vi "base64_decode.vi"(11 "base64":string) -> (3 "string":string)   [LabVIEW 2018, in "hashlib.lvlib"]
doc: "Decodes the <b>Base64</b> data from the <b>base64</b> string input.\n\nRFC 4648\n\nCreated by: Ryan Pacini"
uses:
  hashlib.lvlib
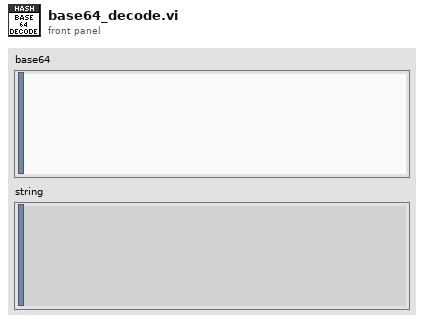
[diagram p1: front panel]
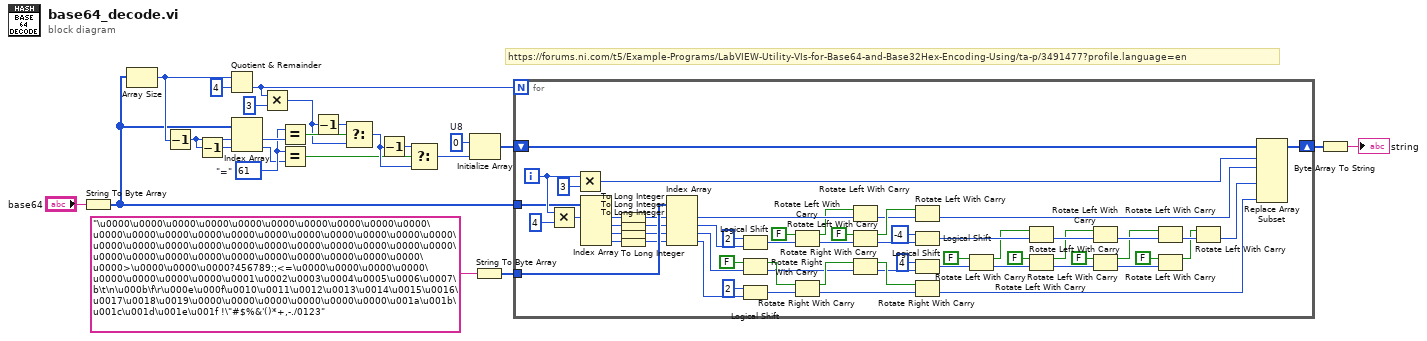
[diagram p0: block diagram]
diagram:
  w11 = u8 61  # "="
  w21 = u8 0  # U8
  # "https://forums.ni.com/t5/Example-Programs/LabVIEW-Utility-VIs-for-Base64-and-Base32Hex-Encoding-Using/ta-p/3491477?profile.language=en"
  n1 = String To Byte Array(string="base64") -> (unsigned byte array=w1:u8[])
  n2 = Array Size(array=w1) -> (size(s)=w18:i32)
  n3 = Decrement(x=w18) -> (x-1=w14:i32)
  n4 = Decrement(x=w14) -> (x-1=w13:i32)
  n5 = Quotient & Remainder(x=w18, y=4) -> (floor(x/y)=w2:i32)  [unwired: 1 out]
  n6 = Index Array(array=w1, index #1=w14, index #2=w13) -> (element #1=w12:u8, element #2=w10:u8)
  n7 = Multiply(x=w2, y=3) -> (x*y=w8:i32)
  n8 = Equal?(x=w11, y=w12) -> (x = y?=w9:bool)
  n9 = Equal?(x=w11, y=w10) -> (x = y?=w4:bool)
  n10 = Decrement(x=w8) -> (x-1=w7:i32)
  n11 = Select(t=w7, s=w9, f=w8) -> (s? t:f=w5:i32)
  n12 = Decrement(x=w5) -> (x-1=w6:i32)
  n13 = Select(t=w6, s=w4, f=w5) -> (s? t:f=w3:i32)
  n14 = Initialize Array(w21, w3) -> (w20:u8[])
  n15 = String To Byte Array(string="\u0000\u0000\u0000\u0000\u0000\u0000\u0000\u0000\u0000\u0000\u0000\u0000\u0000\u0000\u0000\u0000\u0000\u0000\u0000\u0000\u0000\u0000\u0000\u0000\u0000\u0000\u0000\u0000\u0000\u0000\u0000\u0000\u0000\u0000\u0000\u0000\u0000\u0000\u0000\u0000\u0000\u0000\u0000>\u0000\u0000\u0000?456789:;<=\u0000\u0000\u0000\u0000\u0000\u0000\u0000\u0000\u0001\u0002\u0003\u0004\u0005\u0006\u0007\b\t\n\u000b\f\r\u000e\u000f\u0010\u0011\u0012\u0013\u0014\u0015\u0016\u0017\u0018\u0019\u0000\u0000\u0000\u0000\u0000\u0000\u001a\u001b\u001c\u001d\u001e\u001f !\"#$%&'()*+,-./0123") -> (unsigned byte array=w15:u8[])
  n16 = for {
    N: w2 -> [_]
    shift-right: [w37] -> w17
    shift-left: w20 -> [w36]
    tunnel: w1 -> [w79]
    tunnel: w15 -> [w29]
    i -> [w82]
    n17 = Multiply(x=w82, y=4) -> (x*y=w80:i32)
    n18 = Multiply(x=w82, y=3) -> (x*y=w83:i32)
    n19 = Index Array(array=w79, index #1=w80) -> (element #1=w78:u8, element #2=w77:u8, element #3=w76:u8, element #4=w75:u8)  [unwired: 3 in]
    n20 = To Long Integer(number=w78) -> (32bit integer=w28:i32)
    n21 = To Long Integer(number=w77) -> (32bit integer=w27:i32)
    n22 = To Long Integer(number=w76) -> (32bit integer=w26:i32)
    n23 = To Long Integer(number=w75) -> (32bit integer=w25:i32)
    n24 = Index Array(array=w29, index #1=w28, index #2=w27, index #3=w26, index #4=w25) -> (element #1=w74:u8, element #2=w72:u8, element #3=w58:u8, element #4=w59:u8)
    n25 = Logical Shift(y=i16 2, x=w72) -> (x << y=w71:u8)
    n26 = Rotate Right With Carry(2:w58, 3:FALSE ("carry")) -> (0:w55:u8, 1:w57:bool)
    n27 = Logical Shift(y=i16 2, x=w59) -> (x << y=w60:u8)
    n28 = Rotate Left With Carry(2:w71, 3:FALSE ("carry")) -> (0:w68:u8, 1:w67:bool)
    n29 = Rotate Right With Carry(2:w60, 3:w57) -> (0:w53:u8, 1:w56:bool)
    n30 = Rotate Left With Carry(2:w74, 3:w67) -> (0:w65:u8)  [unwired: 1 out]
    n31 = Rotate Left With Carry(2:w68, 3:FALSE ("carry")) -> (0:w62:u8, 1:w66:bool)
    n32 = Rotate Right With Carry(2:w55, 3:w56) -> (0:w46:u8, 1:w54:bool)
    n33 = Rotate Left With Carry(2:w65, 3:w66) -> (0:w64:u8)  [unwired: 1 out]
    n34 = Logical Shift(y=i16 -4, x=w62) -> (x << y=w51:u8)
    n35 = Logical Shift(y=i16 4, x=w46) -> (x << y=w45:u8)
    n36 = Rotate Right With Carry(2:w53, 3:w54) -> (0:w52:u8)  [unwired: 1 out]
    n37 = Rotate Left With Carry(2:w45, 3:FALSE ("carry")) -> (0:w43:u8, 1:w44:bool)
    n38 = Rotate Left With Carry(2:w51, 3:w44) -> (0:w50:u8)  [unwired: 1 out]
    n39 = Rotate Left With Carry(2:w43, 3:FALSE ("carry")) -> (0:w41:u8, 1:w42:bool)
    n40 = Rotate Left With Carry(2:w50, 3:w42) -> (0:w49:u8)  [unwired: 1 out]
    n41 = Rotate Left With Carry(2:w41, 3:FALSE ("carry")) -> (0:w39:u8, 1:w40:bool)
    n42 = Rotate Left With Carry(2:w49, 3:w40) -> (0:w48:u8)  [unwired: 1 out]
    n43 = Rotate Left With Carry(2:w39, 3:FALSE ("carry")) -> (1:w38:bool)  [unwired: 1 out]
    n44 = Rotate Left With Carry(2:w48, 3:w38) -> (0:w35:u8)  [unwired: 1 out]
    n45 = Replace Array Subset(array=w36, new element #1=w64, index #1=w83, new element #2=w35, new element #3=w52) -> (w37:u8[])  [unwired: 2 in]
  }
  n46 = Byte Array To String(unsigned byte array=w17) -> (string=→"string":string)
